vi "booleam2str.vi"(1 "Boolean":bool) -> (0 "Str":string)   [LabVIEW 2014]
doc: "true、false"
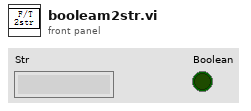
[diagram p1: front panel]
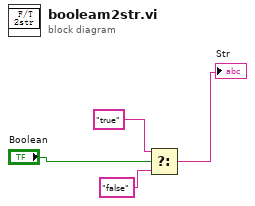
[diagram p0: block diagram]
diagram:
  n1 = Select(t="true", s="Boolean", f="false") -> (s? t:f=→"Str":string)
